vi "Calc K.vi"(7 "Reobserved Array":bool[](array[boolean]), 8 "error in (no error)":errorcluster, 10 "SLAM In":T1) -> (0 "error out":errorcluster, 2 "SLAM Out":T1)   [LabVIEW 2009]
uses:
  Controls/SLAM.ctl
  <vilib>/Analysis/Matrix/Datatypes/RealMatrix.ctl
  <vilib>/Analysis/baseanly.llb/Real A x B.vi
  <vilib>/Analysis/baseanly.llb/Real Inverse Matrix.vi
  <vilib>/Analysis/Matrix/Numeric/Add/Add - RM,RM.vi
  <vilib>/Analysis/7linalg.llb/Real Transpose Matrix.vi
  <vilib>/Analysis/NI_AALBase.lvlib
  <vilib>/Analysis/NI_AALPro.lvlib
  <vilib>/Analysis/Matrix/NI_Matrix.lvlib
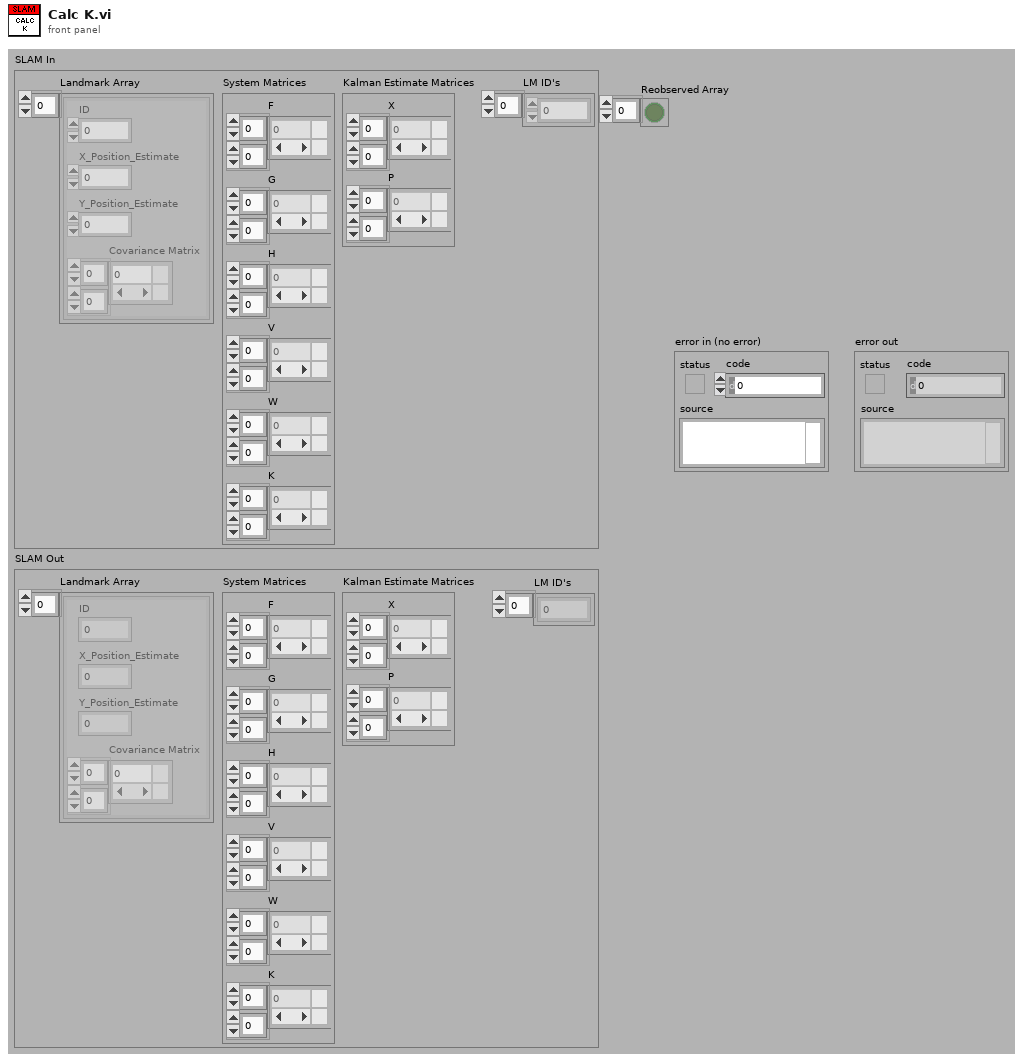
[diagram p1: front panel]
types:
  T1 = typedef "SLAM.ctl" = cluster{"Landmark Array":cluster{"ID":dbl, "X_Position_Estimate":dbl, "Y_Position_Estimate":dbl, "Covariance Matrix":T2}[], "System Matrices":cluster{"F":T2, "G":T2, "H":T2, "V":T2, "W":T2, "K":T2}, "Kalman Estimate Matrices":cluster{"X":T2, "P":T2}, "LM ID's":dbl[]}
  T2 = typedef "NI_Matrix.lvlib/RealMatrix.ctl" = dbl[][]
  T3 = cluster{"F":T2, "G":T2, "H":T2, "V":T2, "W":T2, "K":T2}
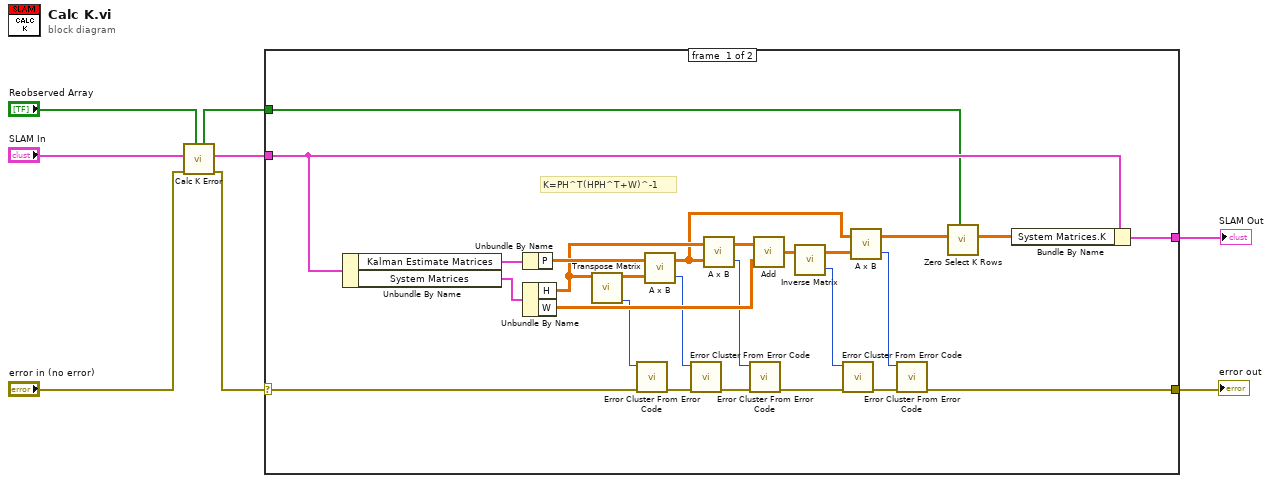
[diagram p0: block diagram]
diagram:
  n1 = call "Calc K Error.vi"("Reobserved Array"="Reobserved Array", "Error In"="error in (no error)", "SLAM In"="SLAM In") -> ("error out"=w2:errorcluster, "SLAM Out"=w4:T1, "Reobserved Array Out"=w5:bool[])  [unwired: 6 in]
  n2 = case shown="No Error" w2 {
    selector: w2 -> [w18 w36]
    tunnel: [w14 w36] -> w8
    tunnel: w4 -> [w13 w35]
    tunnel: [w12 w35] -> w7
    tunnel: w5 -> [w10 _]
    frame #0 {
      # "K=PH^T(HPH^T+W)^-1"
      n3 = Unbundle By Name(w13) -> ("Kalman Estimate Matrices"=w32:cluster{"X":T2, "P":T2}, "System Matrices"=w31:T3)
      n4 = Unbundle By Name(w32) -> ("P"=w33:T2)
      n5 = Unbundle By Name(w31) -> ("H"=w30:T2, "W"=w28:T2)
      n6 = call-poly <vilib>:"Transpose Matrix.vi"("Input Matrix"=w30) -> ("error"=w24:i32, "Matrix Transpose"=w34:T2)  [unwired: 9 in]
      n7 = call <vilib>:"Error Cluster From Error Code.vi"("error in (no error)"=w18, "error code (0)"=w24) -> ("error out"=w23:errorcluster)  [unwired: 7 in]
      n8 = call-poly <vilib>:"A x B.vi"("B"=w34, "A"=w33) -> ("error"=w22:i32, "A x B"=w26:T2)
      n9 = call <vilib>:"Error Cluster From Error Code.vi"("error in (no error)"=w23, "error code (0)"=w22) -> ("error out"=w17:errorcluster)  [unwired: 7 in]
      n10 = call-poly <vilib>:"A x B.vi"("B"=w26, "A"=w30) -> ("error"=w21:i32, "A x B"=w27:T2)
      n11 = call <vilib>:"Error Cluster From Error Code.vi"("error in (no error)"=w17, "error code (0)"=w21) -> ("error out"=w16:errorcluster)  [unwired: 7 in]
      n12 = call-poly <vilib>:"Add.vi"("Real Matrix B"=w28, "Real Matrix A"=w27) -> ("A + B"=w29:T2)
      n13 = call-poly <vilib>:"Inverse Matrix.vi"("Input Matrix"=w29) -> ("error"=w20:i32, "Inverse Matrix"=w25:T2)  [unwired: 1 in]
      n14 = call <vilib>:"Error Cluster From Error Code.vi"("error in (no error)"=w16, "error code (0)"=w20) -> ("error out"=w15:errorcluster)  [unwired: 7 in]
      n15 = call-poly <vilib>:"A x B.vi"("B"=w25, "A"=w26) -> ("error"=w19:i32, "A x B"=w11:T2)
      n16 = call <vilib>:"Error Cluster From Error Code.vi"("error in (no error)"=w15, "error code (0)"=w19) -> ("error out"=w14:errorcluster)  [unwired: 7 in]
      n17 = call "Zero Select K Rows.vi"("Reobserved Array"=w10, "K In"=w11) -> ("K Out"=w9:T2)  [unwired: 9 in]
      n18 = Bundle By Name(cluster=w13, "System Matrices.K"=w9) -> (w12:T1)
    }
    frame #1 {
    }
  }
  "error out" <- w8
  "SLAM Out" <- w7
